vi "LINXSoundInput(SubVI).vi"(6 "Duration (ms)":u32, 9 "Channel":u8, 10 "Enter frequency:":dbl, 11 "VISA Refnum in":refnum<visa-resource-name>) -> ()   [LabVIEW 2014]
uses:
  <vilib>/MakerHub/LINX/LMH-LINX.lvlib
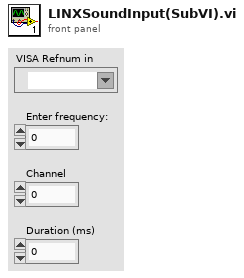
[diagram p1: front panel]
types:
  T1 = typedef "LMH-LINX.lvlib/LINX Ref.ctl" = cluster{"IO":T2, "Interface":T3, "LINX Device Config":T4}
  T2 = typedef "LMH-LINX.lvlib/Platform.ctl" = enum16{"Remote", "Local"}
  T3 = typedef "LMH-LINX.lvlib/Interface.ctl" = enum16{"Serial", "TCP"}
  T4 = typedef "LMH-LINX.lvlib/Device.lvlib/LINX Device Config.ctl" = cluster{"Interface":T3, "COM Port":refnum<visa-resource-name>, "TCP Configuration":T5, "Device Family":u8, "Device ID":u8, "Device Name":string, "TCP Ref":refnum<k5>, "Channels":T6}
  T5 = typedef "LMH-LINX.lvlib/Device.lvlib/TCP Config.ctl" = cluster{"IP Address":string, "Port":u16}
  T6 = typedef "LMH-LINX.lvlib/Channels.ctl" = cluster{"DI":u8[], "DO":u8[], "AI":u8[], "AO":u8[], "PWM":u8[], "QE":u8[], "UART":u8[], "I2C 2":u8[], "SPI":u8[], "CAN":u8[], "Servo":u8[], "AI Ref (V)":dbl, "AI Resolution (Bits)":u8, "AO Ref (V)":dbl, "AO Resolution (Bits)":u8}
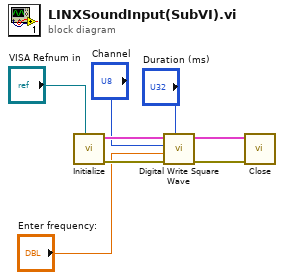
[diagram p0: block diagram]
diagram:
  n1 = call <vilib>:"Initialize.vi"("Serial Port"="VISA Refnum in") -> ("Error Out"=w6:errorcluster, "LINX Resource"=w5:T1)  [unwired: 8 in, 1 out]
  n2 = call <vilib>:"Digital Write Square Wave.vi"("Duration (ms)"="Duration (ms)", "Error In"=w6, "Frequency (Hz)"="Enter frequency:", "Channel"="Channel", "LINX Resource"=w5) -> ("Error Out"=w8:errorcluster, "LINX Resource"=w7:T1)  [unwired: 5 in]
  n3 = call <vilib>:"Close.vi"("Error In"=w8, "LINX Resource"=w7) -> ()  [unwired: 9 in, 1 out]
